vi "Set WIFI Port.vi"(8 "Error In":errorcluster, 10 "Port":u16, 11 "LINX Device Config":T1) -> (0 "Error Out":errorcluster, 3 "LINX Device Config":T1)   [LabVIEW 2011, in "LMH-LINX.lvlib" / "Device.lvlib"]
doc: "Set the LINX device's WIFI port."
uses:
  Device.lvlib
  Type Defs/LINX Device Config.ctl
  Type Defs/Interface.ctl
  Type Defs/TCP Config.ctl
  Type Defs/Channels.ctl
  Type Defs/Error Type.ctl
  LMH-LINX.lvlib
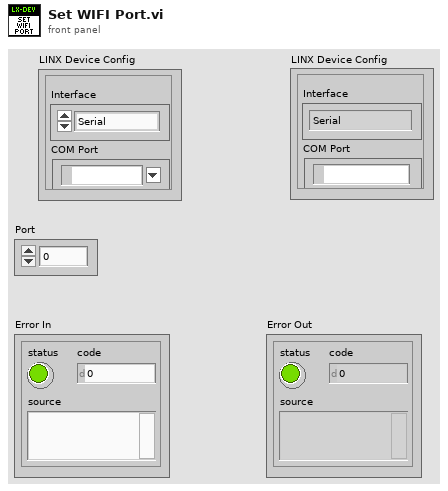
[diagram p1: front panel]
types:
  T1 = typedef "LMH-LINX.lvlib/Device.lvlib/LINX Device Config.ctl" = cluster{"Interface":T2, "COM Port":refnum<visa-resource-name>, "TCP Configuration":T3, "Device Family":u8, "Device ID":u8, "Device Name":string, "TCP Ref":refnum<k5>, "Channels":T4}
  T2 = typedef "LMH-LINX.lvlib/Interface.ctl" = enum16{"Serial", "TCP"}
  T3 = typedef "LMH-LINX.lvlib/Device.lvlib/TCP Config.ctl" = cluster{"IP Address":string, "Port":u16}
  T4 = typedef "LMH-LINX.lvlib/Channels.ctl" = cluster{"DI":u8[], "DO":u8[], "AI":u8[], "AO":u8[], "PWM":u8[], "QE":u8[], "UART":u8[], "I2C 2":u8[], "SPI":u8[], "CAN":u8[], "Servo":u8[], "AI Ref (V)":dbl, "AO Ref (V)":dbl, "AO Resolution (Bits)":u8}
  T5 = typedef "LMH-LINX.lvlib/Error Type.ctl" = enum16{"Unknown", "Timeout", "Corrupt Return Packet", "Unable To Connect", "Command Not Supported", "Channel DNE", "Invalid COM Config", "Firmware Version Mismatch", "myRIO Support", "CMD Specific Error"}
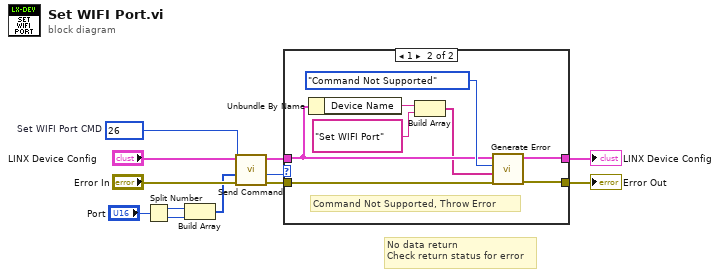
[diagram p0: block diagram]
diagram:
  w8 = u16 26  # Set WIFI Port CMD
  # "No data return\nCheck return status for error"
  n1 = Split Number(x="Port") -> (hi(x)=w11:u8, lo(x)=w10:u8)
  n2 = Build Array(w11, w10) -> (w2:u8[])
  n3 = call "Send Command.vi"("Error In"="Error In", "ARGS"=w2, "CMD"=w8, "LINX Device Config"="LINX Device Config") -> ("Error Out"=w3:errorcluster, "Status"=w1:u8, "LINX Device Config"=w5:T1)  [unwired: 4 in, 1 out]
  n4 = case shown="1" w1 {
    tunnel: [w13 w20] -> w6
    tunnel: w5 -> [w13 w16]
    tunnel: [w14 w21] -> w4
    tunnel: w3 -> [w14 w22]
    frame 0, Default {
      # "Status OK, Process Data"
    }
    frame 1 {
      # "Command Not Supported, Throw Error"
      n5 = Unbundle By Name(w16) -> ("Device Name"=w17:string)
      n6 = Build Array(w17, "Set WIFI Port") -> (w15:string[])
      n7 = call "Generate Error.vi"("Error In"=w22, "Arguments"=w15, "Error Type"=Error_Type."Command Not Supported", "LINX Device Config"=w16) -> ("Error Out"=w21:errorcluster, "LINX Device Config"=w20:T1)  [unwired: 6 in]
    }
  }
  "Error Out" <- w4
  "LINX Device Config" <- w6
